vi "WriteMultipleDigitalOutputs.vi"(8 "error in (no error)":errorcluster, 10 "data":bool[](array[boolean]), 11 "DigitalOutput_Simulation In":refnum<class "TesteractHAL_DigitalOutput_Simulation.lvclass">) -> (0 "error out":errorcluster, 3 "DigitalOutput_Simulation Out":refnum<class "TesteractHAL_DigitalOutput_Simulation.lvclass">)   [LabVIEW 2017, in "TesteractHAL_DigitalOutput_Simulation.lvlib" / "TesteractHAL_DigitalOutput_Simulation.lvclass"]
doc: "Write multiple digital signals using an array of booleans."
uses:
  TesteractHAL_DigitalOutput_Simulation.lvclass
  TesteractHAL_DigitalOutput_Simulation.lvclass/TesteractHAL_DigitalOutput_Simulation.ctl
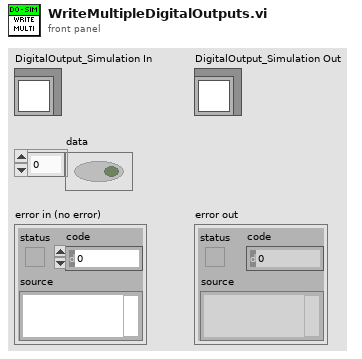
[diagram p1: front panel]
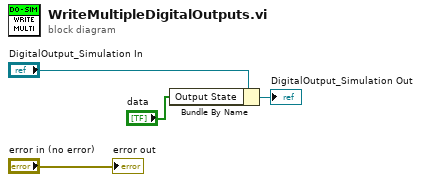
[diagram p0: block diagram]
diagram:
  n1 = Bundle By Name(cluster="DigitalOutput_Simulation In", "Output State"="data") -> (→"DigitalOutput_Simulation Out":refnum<class "TesteractHAL_DigitalOutput_Simulation.lvclass">)
  "error out" <- "error in (no error)"
